vi "Intake.vi"(8 "error in (no error)":errorcluster, 9 "Out":bool, 10 "In":bool, 11 "Cargo PacBot in":refnum<class "Cargo PacBot.lvclass">) -> (0 "error out":errorcluster, 3 "Cargo PacBot out":refnum<class "Cargo PacBot.lvclass">)   [LabVIEW 2018, in "Cargo.lvlib" / "Cargo PacBot.lvclass"]
doc: "Use this VI to operate the intake"
uses:
  Cargo PacBot.lvclass
  C:/Users/Public/Documents/2019DeepSpace/Classes/Cargo/Cargo.lvclass
  <vilib>/Rock Robotics/WPI/ThirdParty/Phoenix-LabVIEW/Motor Controller/Controls/CTRE_Phoenix_MotorControl_ControlMode.ctl
  Cargo PacBot.lvclass/Cargo PacBot.ctl
  Cargo.lvclass
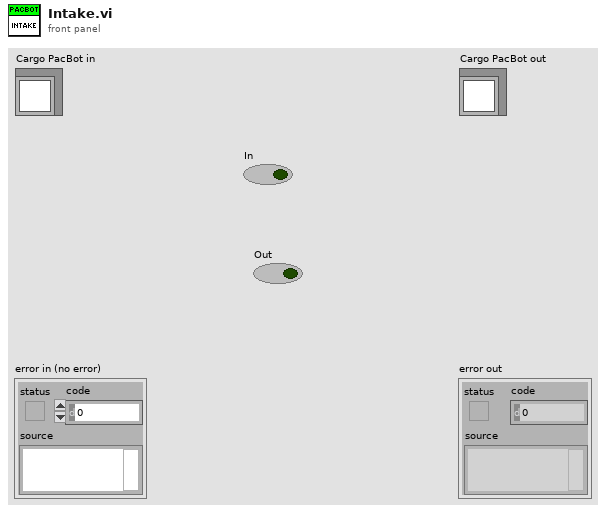
[diagram p1: front panel]
types:
  T1 = typedef "CTRE_Phoenix_MotorControl_ControlMode.ctl" = u16
  T2 = typedef "Cargo.lvlib/Cargo.lvclass/Cargo States.ctl" = enum16{"Off", "Intake Full", "Intake Idle", "Output Full"}
  T3 = typedef "WPI_MotorControlDeviceRef.ctl" = cluster{"DeviceStatus":errorcluster, "Type":T4, "PWM":cluster{"PWM Channel":T5, "DeadBand":T6}, "CAN":cluster{"Device Number":u8, "SetOutput VI Ref":variant, "GetOutput VI Ref":variant, "Enable VI Ref":variant, "Disable VI Ref":variant, "Data":variant}, "Invert":bool, "DIO PWM":cluster{"PWM \"Enable\" Channel":T5, "DIOChannel":T7, "PWM Rate":dbl}}
  T4 = typedef "WPI_MotorControlType.ctl" = enum16{"PWM", "CAN", "DIO PWM"}
  T5 = typedef "FPGA_DIOPWMChannel.ctl" = enum8{"PWM 0", "PWM 1", "PWM 2", "PWM 3", "PWM 4", "PWM 5", "PWM 6", "PWM 7", "PWM 8", "PWM 9", "PWM MXP 0", "PWM MXP 1", "PWM MXP 2", "PWM MXP 3", "PWM MXP 4", "PWM MXP 5", "PWM MXP 6", "PWM MXP 7", "PWM MXP 8", "PWM MXP 9", "Invalid"}
  T6 = typedef "WPI_PWMDeadband.ctl" = cluster{"Name":string, "maxPositivePwm":i32, "minPositivePwm":i32, "centerPwm":i32, "maxNegativePwm":i32, "minNegativePwm":i32, "angularRange":u16}
  T7 = typedef "FPGA_DIOChannel.ctl" = enum8{"DIO 0", "DIO 1", "DIO 2", "DIO 3", "DIO 4", "DIO 5", "DIO 6", "DIO 7", "DIO 8", "DIO 9", "DIO MXP 0", "DIO MXP 1", "DIO MXP 2", "DIO MXP 3", "DIO MXP 4", "DIO MXP 5", "DIO MXP 6", "DIO MXP 7", "DIO MXP 8", "DIO MXP 9", "DIO MXP 10", "DIO MXP 11", "DIO MXP 12", "DIO MXP 13", "DIO MXP 14", "DIO MXP 15", "SPI Port CS1", "SPI Port CS2", "SPI Port CS3", "SPI Port MISO", "SPI Port MOSI", "Invalid"}
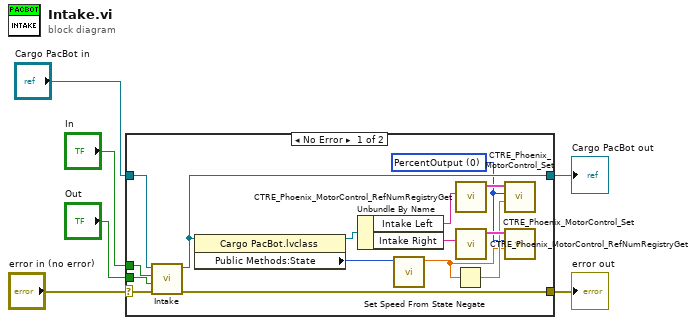
[diagram p0: block diagram]
diagram:
  n1 = case shown="No Error" "error in (no error)" {
    selector: "error in (no error)" -> [w20 w23]
    tunnel: [w21 w23] -> w1
    tunnel: [w12 w22] -> w3
    tunnel: "Cargo PacBot in" -> [w14 w22]
    tunnel: "In" -> [w11 _]
    tunnel: "Out" -> [w10 _]
    frame No Error {
      w7 = T1 0 items=["PercentOutput"=0, "Position"=1, "Velocity"=2, "Current"=3, "Follower"=5, "MotionProfile"=6, "MotionMagic"=7, "MotionProfileArc"=10, "Disabled"=15] ("Control Mode")
      n2 = call-parent "Intake.vi"("error in (no error)"=w20, "Out"=w10, "In"=w11, "Cargo in"=w14) -> ("error out"=w21:errorcluster, "Cargo out"=w12:refnum<class "Cargo PacBot.lvclass">)  [unwired: 6 in]
      n3 = property class="Cargo PacBot.lvclass"(reference=w12) -> (reference out=w13:refnum<class "Cargo PacBot.lvclass">, "Public Methods:State"=w15:T2)  [unwired: 1 in, 1 out]
      n4 = Unbundle By Name(w13) -> ("Intake Left"=w19:string, "Intake Right"=w18:string)
      n5 = call "Set Speed From State.vi"("Public Methods:State"=w15) -> ("Output"=w8:dbl)  [unwired: 10 in]
      n6 = Negate(x=w8) -> (-x=w9:dbl)
      n7 = call <vilib>:"CTRE_Phoenix_MotorControl_RefNumRegistryGet.vi"("refnum name"=w19) -> ("PhoenixMotorControlDevRef"=w17:T3)  [unwired: 9 in, 1 out]
      n8 = call <vilib>:"CTRE_Phoenix_MotorControl_RefNumRegistryGet.vi"("refnum name"=w18) -> ("PhoenixMotorControlDevRef"=w16:T3)  [unwired: 9 in, 1 out]
      n9 = call <vilib>:"CTRE_Phoenix_MotorControl_Set.vi"("Output"=w9, "Control Mode"=w7, "PhoenixMotorControlDevRef"=w17) -> ()  [unwired: 7 in, 2 out]
      n10 = call <vilib>:"CTRE_Phoenix_MotorControl_Set.vi"("Output"=w8, "Control Mode"=w7, "PhoenixMotorControlDevRef"=w16) -> ()  [unwired: 7 in, 2 out]
    }
    frame Error {
    }
  }
  "error out" <- w1
  "Cargo PacBot out" <- w3
